vi "FG Reset Encoder Position.vi"(1 "FG Action":T1, 2 "Reset Encoder?":bool) -> (0 "Reset Reset Encoder?":bool)   [LabVIEW 2009]
uses:
  Actions for FG's.ctl
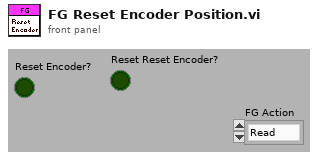
[diagram p1: front panel]
types:
  T1 = typedef "Actions for FG's.ctl" = enum16{"Read", "Write"}
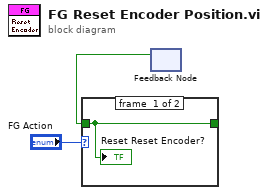
[diagram p0: block diagram]
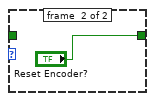
[diagram p2: hidden frame]
diagram:
  n1 = feedback #1() -> (w1:bool)  [unwired: 1 in]
  n2 = case shown="\"Read\", Default" "FG Action" {
    tunnel: [w4 "Reset Encoder?"] -> w2
    tunnel: w1 -> [w4 _]
    frame #0 {
      "Reset Reset Encoder?" <- w4
    }
    frame #1 {
    }
  }
